vi "ReadMercuryVISA.vi"() -> ()   [LabVIEW 2014]
panel:
  out "Numeric":dbl
  out "error out":errorcluster
  out "String":string
  in  "error in (no error)":errorcluster
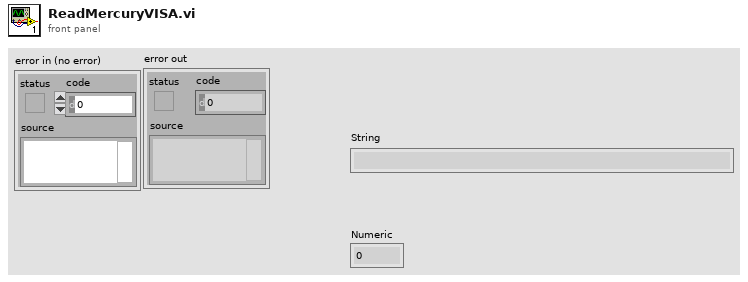
[diagram p1: front panel]
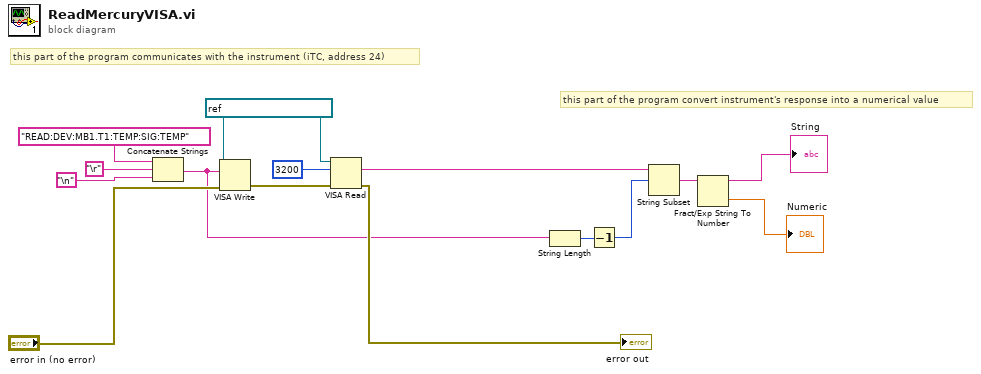
[diagram p0: block diagram]
diagram:
  w12 = refnum<visa-resource-name> "GPIB0::24::1::INSTR" ("VISA resource name")
  # "this part of the program convert instrument's response into a numerical value"
  # "this part of the program communicates with the instrument (iTC, address 24)"
  n1 = Concatenate Strings("READ:DEV:MB1.T1:TEMP:SIG:TEMP" ("string"), "\r", "\n") -> (w6:string)
  n2 = VISA Write(VISA resource name=w12, write buffer=w6, error in (no error)="error in (no error)") -> (error out=w13:errorcluster)  [unwired: 2 out]
  n3 = VISA Read(VISA resource name=w12, byte count=3200, error in (no error)=w13) -> (read buffer=w5:string, error out=→"error out":errorcluster)  [unwired: 2 out]
  n4 = String Length(string=w6) -> (length=w2:i32)
  n5 = Decrement(x=w2) -> (x-1=w1:i32)
  n6 = String Subset(string=w5, offset (0)=w1) -> (substring=w4:string)  [unwired: 1 in]
  "String" <- w4
  n7 = Fract/Exp String To Number(string=w4) -> (number=→"Numeric":dbl)  [unwired: 3 in, 1 out]
